vi "Release.vi"(8 "error in (no error)":errorcluster, 11 "EStop Source in":refnum<class "EStop Source.lvclass">) -> (0 "error out":errorcluster)   [LabVIEW 2020, in "VolatusControl.lvlib" / "EStop Source.lvclass"]
uses:
  EStop Source.lvclass
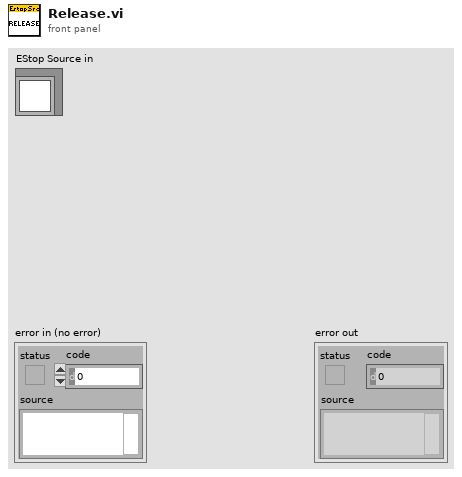
[diagram p1: front panel]
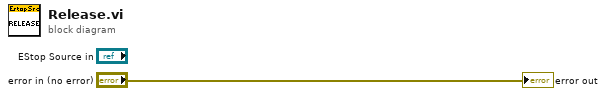
[diagram p0: block diagram]
diagram:
  "error out" <- "error in (no error)"
